vi "Read_SR7265lockIn.vi"() -> ()   [LabVIEW 2015]
panel:
  out "String":string
  out "error out":errorcluster
  in  "error in (no error)":errorcluster
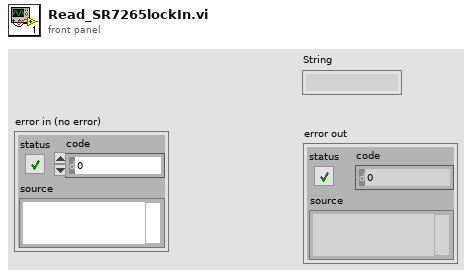
[diagram p1: front panel]
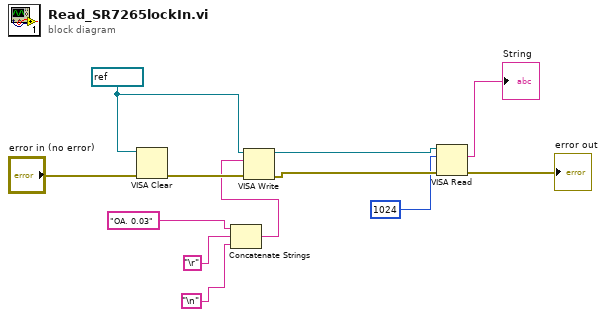
[diagram p0: block diagram]
diagram:
  w10 = refnum<visa-resource-name> "7265" ("VISA resource name")
  n1 = VISA Clear(VISA resource name=w10, error in (no error)="error in (no error)") -> (error out=w11:errorcluster)  [unwired: 1 out]
  n2 = Concatenate Strings("OA. 0.03", "\r", "\n") -> (w6:string)
  n3 = VISA Write(VISA resource name=w10, write buffer=w6, error in (no error)=w11) -> (VISA resource name out=w5:refnum<visa-resource-name>, error out=w4:errorcluster)  [unwired: 1 out]
  n4 = VISA Read(VISA resource name=w5, byte count=1024, error in (no error)=w4) -> (read buffer=→"String":string, error out=→"error out":errorcluster)  [unwired: 2 out]
